vi "Tag Settings Window.vi"(8 "Error In":errorcluster, 11 "Database Connection":refnum<k7>) -> (0 "Error Out":errorcluster)   [LabVIEW 2019]
panel:
  in  "Link Tag Button":bool
  in  "Edit Tag Button":bool
  in  "Remove Tag Button":bool
  in  "Add Tag Button":bool
  in  "Exit Button":bool
  in  "Tag List":i32(listbox) caption="Tags for Device USB-6008-1:"
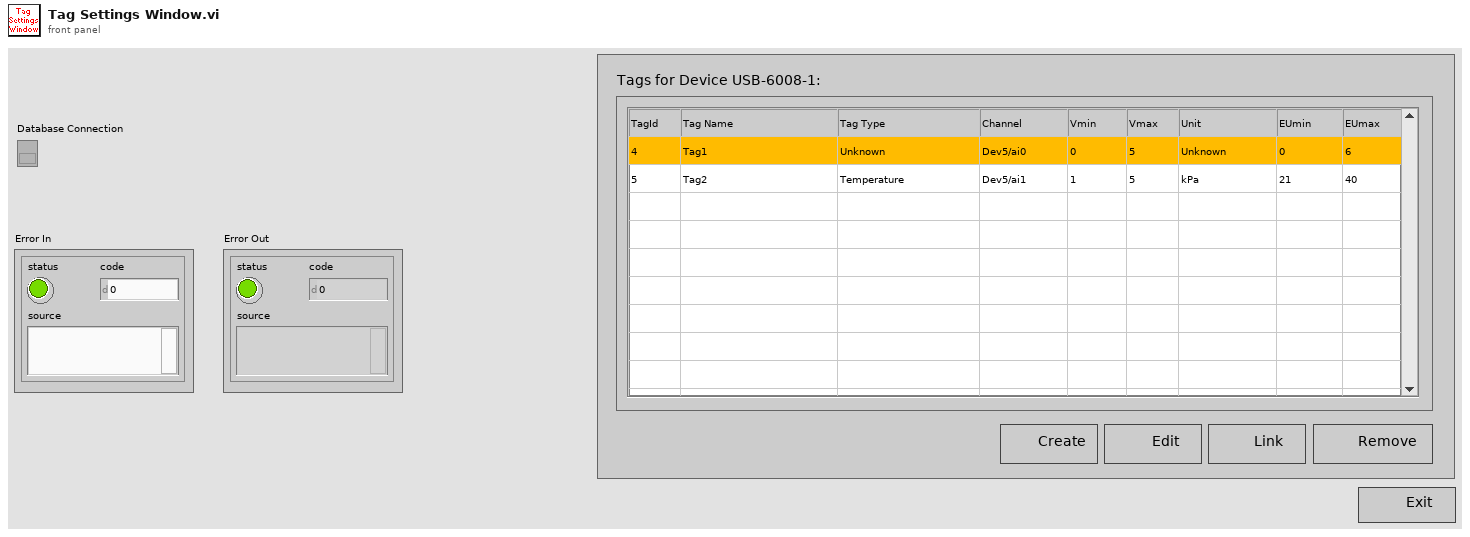
[diagram p1: front panel]
types:
  T1 = typedef "Device Settings.ctl" = cluster{"Device Type":string, "Device Name":string, "DAQmx Name":tag, "Terminal Wiring":i32}
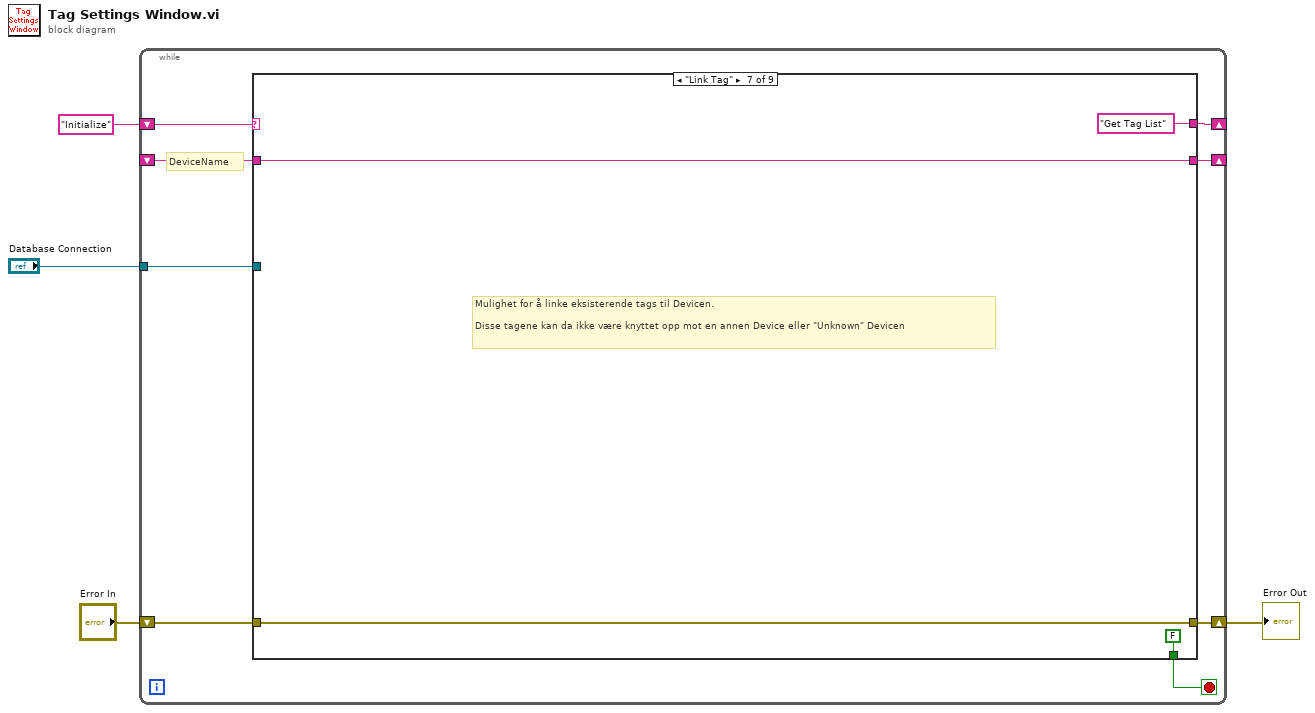
[diagram p0: block diagram]
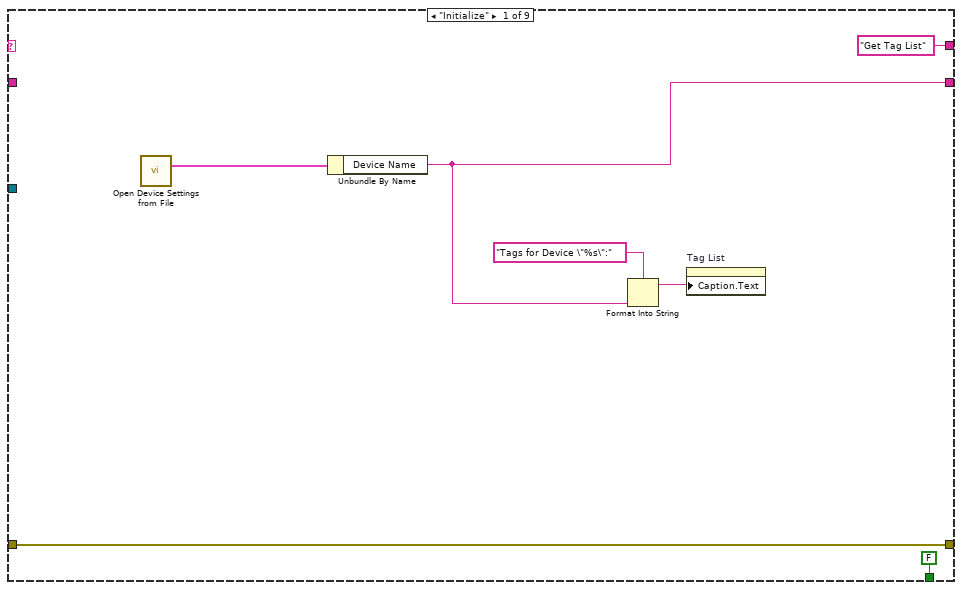
[diagram p2: hidden frame]
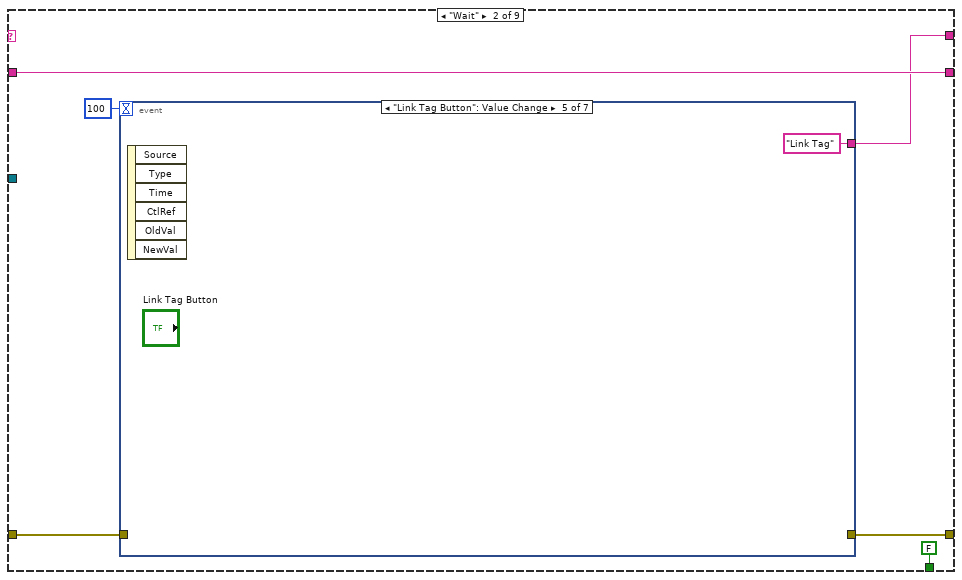
[diagram p3: hidden frame]
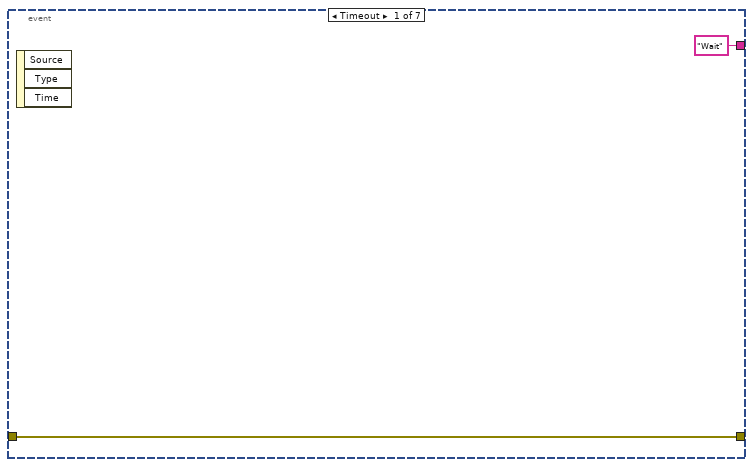
[diagram p4: hidden frame]
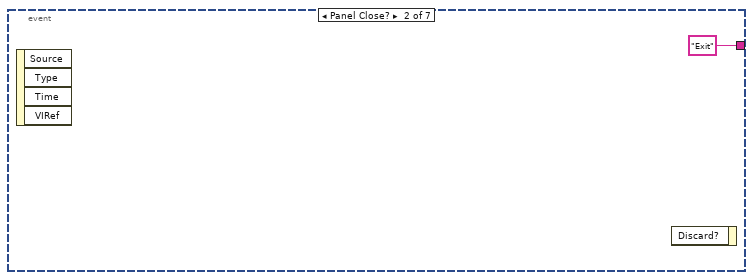
[diagram p5: hidden frame]
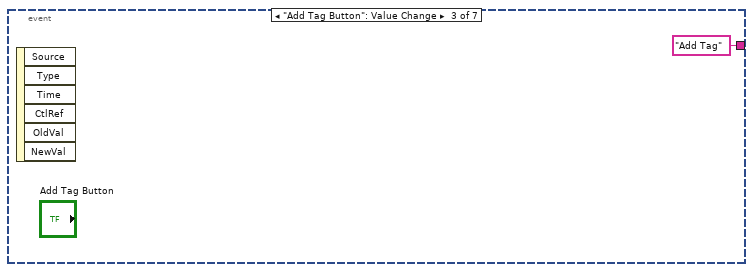
[diagram p6: hidden frame]
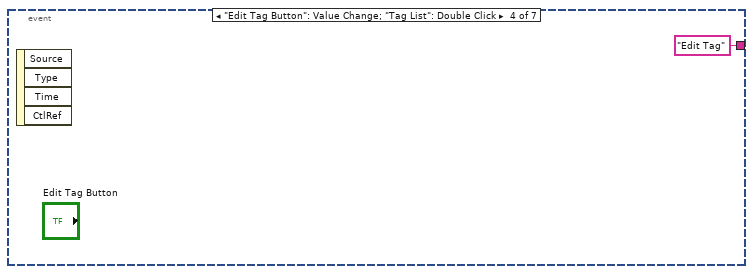
[diagram p7: hidden frame]
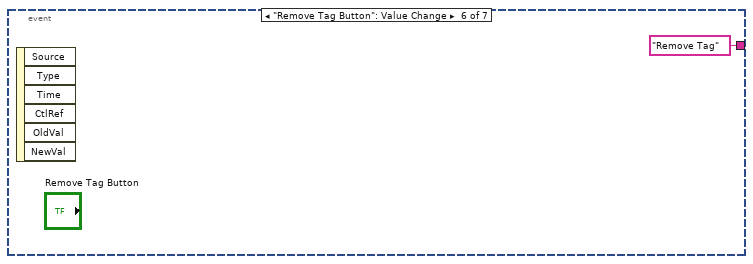
[diagram p8: hidden frame]
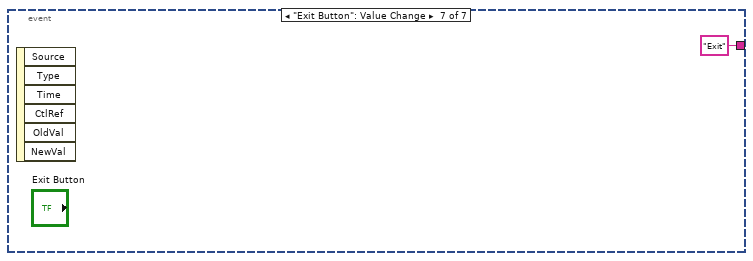
[diagram p9: hidden frame]
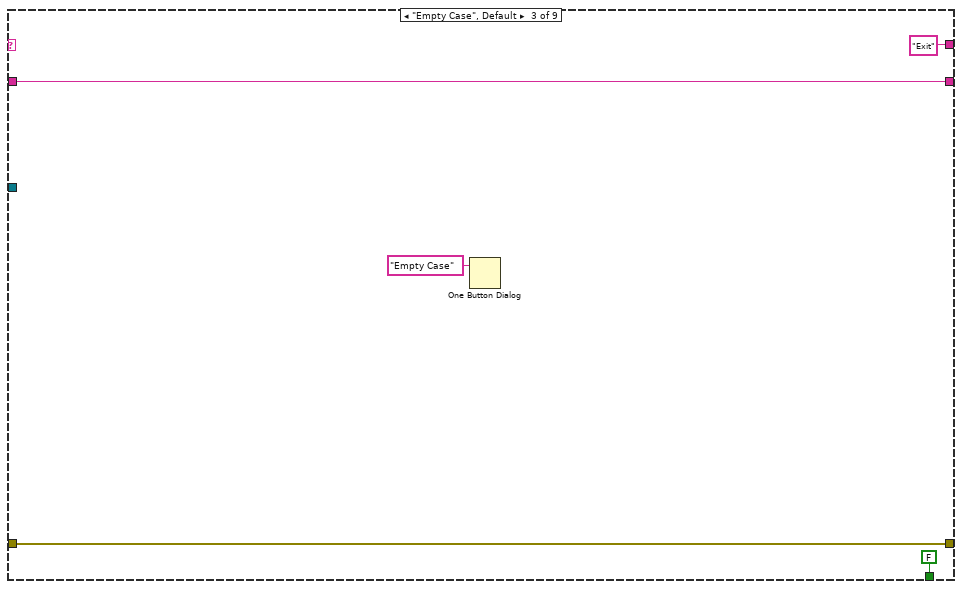
[diagram p10: hidden frame]
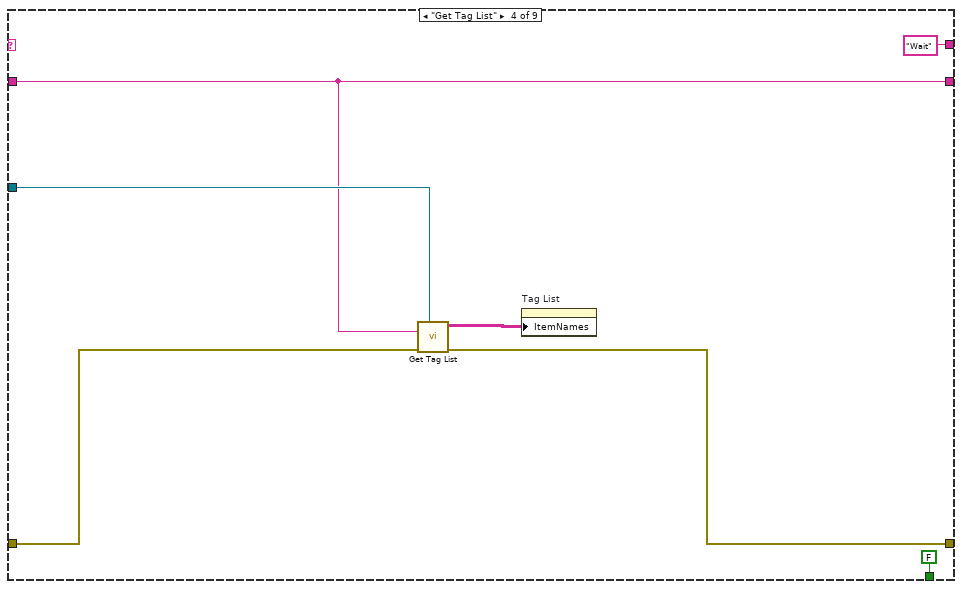
[diagram p11: hidden frame]
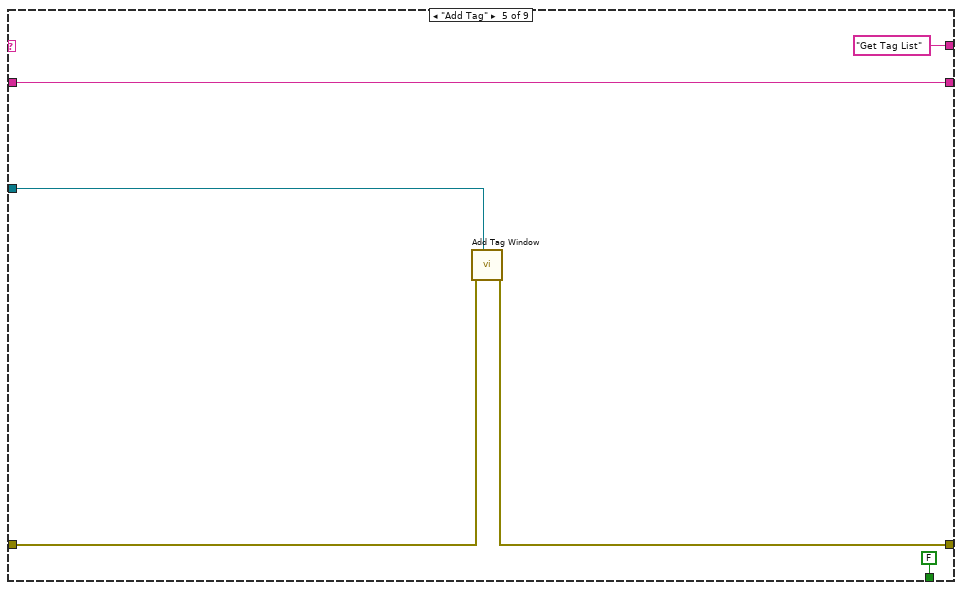
[diagram p12: hidden frame]
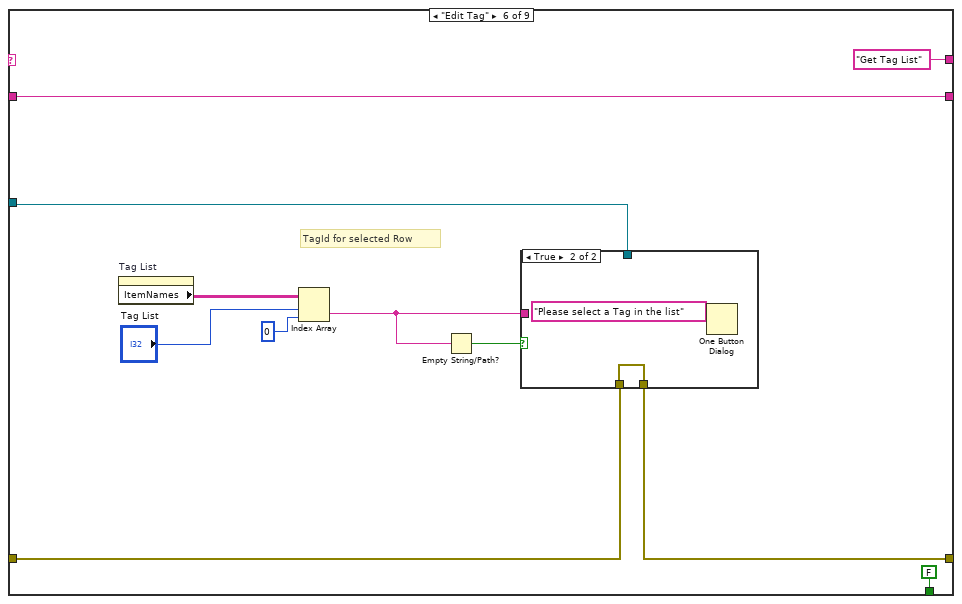
[diagram p13: hidden frame]
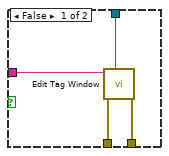
[diagram p14: hidden frame]
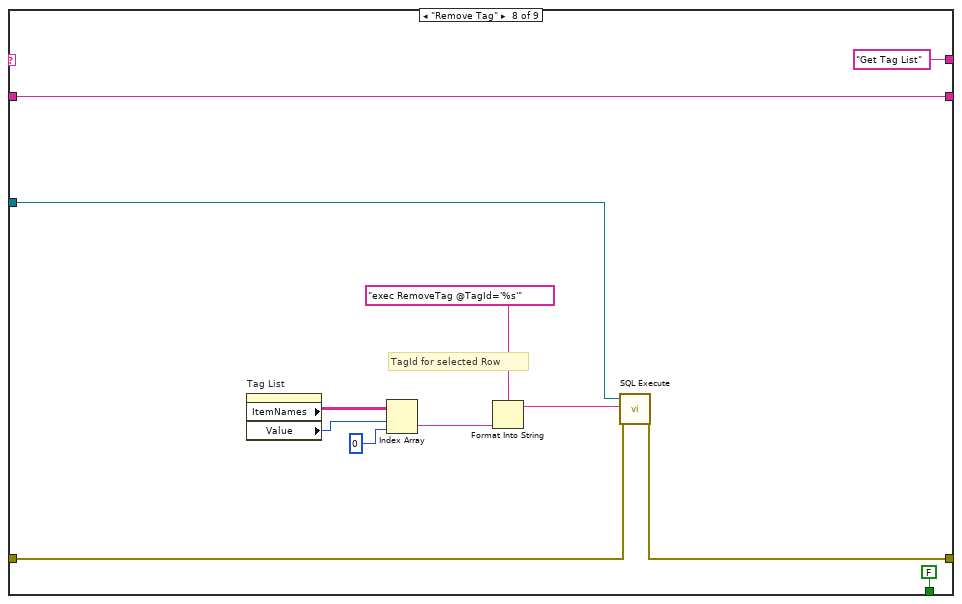
[diagram p15: hidden frame]
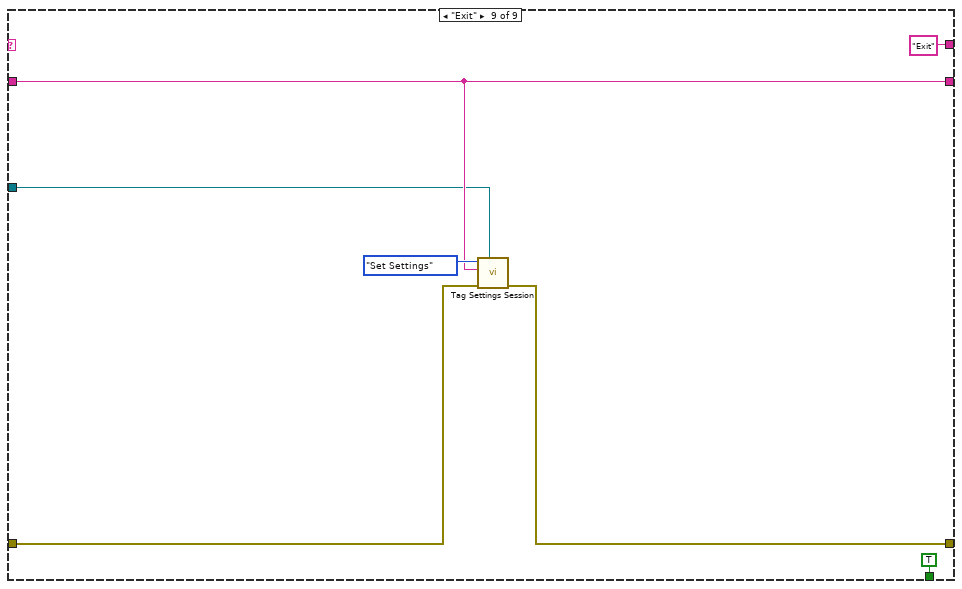
[diagram p16: hidden frame]
diagram:
  n1 = while {
    shift-right: [w8] -> _
    shift-left: "Initialize" ("key") -> [w12]
    shift-right: [w9] -> _
    shift-left: _ -> [w11]
    shift-right: [w6] -> w2
    shift-left: "Error In" -> [w10]
    tunnel: "Database Connection" -> [w5]
    stop <- w7 stop-if-true
    # "DeviceName"
    n2 = case shown="\"Link Tag\"" w12 {
      tunnel: w11 -> [_ w24 w35 w40 w49 w60 w70 w82 w86]
      tunnel: w10 -> [w17 w21 w36 w39 w48 w57 w69 w80 w88]
      tunnel: [w14 w24 w35 w40 w49 w60 w70 w82 w86] -> w9
      tunnel: ["Get Tag List" ("key") w23 "Exit" ("key") "Wait" ("key") "Get Tag List" ("key") "Get Tag List" ("key") "Get Tag List" ("key") "Get Tag List" ("key") "Exit" ("key")] -> w8
      tunnel: [FALSE FALSE FALSE FALSE FALSE FALSE FALSE FALSE TRUE] -> w7
      tunnel: [w17 w20 w36 w42 w47 w56 w69 w79 w87] -> w6
      tunnel: w5 -> [_ _ _ w43 w46 w58 _ w81 w85]
      frame "Initialize" {
        n3 = call "Open Device Settings from File.vi"() -> ("Device Settings"=w16:T1)  [unwired: 14 in, 1 out]
        n4 = Unbundle By Name(w16) -> ("Device Name"=w14:string)
        n5 = Format Into String(format string="Tags for Device \"%s\":", w14) -> (resulting string=w13:string)  [unwired: 2 in, 1 out]
        n6 = property on="Tag List" class="MCListbox (strict)"("Caption.Text"=w13) -> ()  [unwired: 2 in, 2 out]
      }
      frame "Wait" {
        n7 = event shown="[4] \"Link Tag Button\": Value Change" {
          selector: _ -> [_ _ _ _ _ _ _]
          dyn-events: _ -> [_ _ _ _ _ _ _]
          timeout: 100 -> [_ _ _ _ _ _ _]
          tunnel: ["Wait" ("key") "Exit" ("key") "Add Tag" ("key") "Edit Tag" ("key") "Link Tag" ("key") "Remove Tag" ("key") "Exit" ("key")] -> w23
          tunnel: w21 -> [w26 _ _ _ _ _ _]
          tunnel: [w26 _ _ _ _ _ _] -> w20
          event Timeout {
            n8 = event-data() -> ()  [unwired: 1 in, 3 out]
          }
          event Panel Close? {
            n9 = event-data() -> ()  [unwired: 1 in, 4 out]
            n10 = event-data() -> ()  [unwired: 2 in, 1 out]
          }
          event "Add Tag Button": Value Change {
            n11 = event-data() -> ()  [unwired: 1 in, 6 out]
          }
          event "Edit Tag Button": Value Change; "Tag List": Double Click {
            n12 = event-data() -> ()  [unwired: 1 in, 4 out]
          }
          event "Link Tag Button": Value Change {
            n13 = event-data() -> ()  [unwired: 1 in, 6 out]
          }
          event "Remove Tag Button": Value Change {
            n14 = event-data() -> ()  [unwired: 1 in, 6 out]
          }
          event "Exit Button": Value Change {
            n15 = event-data() -> ()  [unwired: 1 in, 6 out]
          }
        }
      }
      frame "Empty Case", Default {
        n16 = One Button Dialog(message="Empty Case") -> ()  [unwired: 1 in, 1 out]
      }
      frame "Get Tag List" {
        n17 = call "Get Tag List.vi"("Database Connection"=w43, "Error In"=w39, "DeviceName"=w40) -> ("Error Out"=w42:errorcluster, "Tag List"=w41:string[][])  [unwired: 7 in]
        n18 = property on="Tag List" class="MCListbox (strict)"("ItemNames"=w41) -> ()  [unwired: 2 in, 2 out]
      }
      frame "Add Tag" {
        n19 = call "Add Tag Window.vi"("Database Connection"=w46, "Error In"=w48) -> ("Error Out"=w47:errorcluster)  [unwired: 9 in]
      }
      frame "Edit Tag" {
        # "TagId for selected Row"
        n20 = property on="Tag List" class="MCListbox (strict)"() -> ("ItemNames"=w59:string[][])  [unwired: 2 in, 2 out]
        n21 = Index Array "Index Array"(array=w59, index (row)="Tag List", index (col)=0 ("index (row)")) -> (element=w53:string)
        n22 = Empty String/Path?(string/path=w53) -> (empty?=w52:bool)
        n23 = case shown="True" w52 {
          tunnel: w58 -> [w66 _]
          tunnel: w57 -> [w65 w68]
          tunnel: [w64 w68] -> w56
          tunnel: w53 -> [w63 _]
          frame False {
            n24 = call "Edit Tag Window.vi"("Database Connection"=w66, "Error In"=w65, "TagId"=w63) -> ("Error Out"=w64:errorcluster)  [unwired: 8 in]
          }
          frame True {
            n25 = One Button Dialog(message="Please select a Tag in the list") -> ()  [unwired: 1 in, 1 out]
          }
        }
      }
      frame "Link Tag" {
        # "Mulighet for å linke eksisterende tags til Devicen.\n\nDisse tagene kan da ikke være knyttet opp mot en annen Device eller \"Unknown\" Devicen"
      }
      frame "Remove Tag" {
        # "TagId for selected Row"
        n26 = property on="Tag List" class="MCListbox (strict)"() -> ("ItemNames"=w77:string[][], "Value"=w76:i32)  [unwired: 2 in, 2 out]
        n27 = Index Array "Index Array"(array=w77, index (row)=w76, index (col)=0 ("index (row)")) -> (element=w75:string)
        n28 = Format Into String "Format Into String"(format string="exec RemoveTag @TagId='%s'", w75) -> (resulting string=w73:string)  [unwired: 2 in, 1 out]
        n29 = call <vilib>:"SQL Execute.vi"("Connection In"=w81, "SQL Query"=w73, "Error in (no error)"=w80) -> ("Error out"=w79:errorcluster)  [unwired: 15 in, 1 out]
      }
      frame "Exit" {
        n30 = call "Tag Settings Session.vi"("Database Connection"=w85, "Error In"=w88, "DeviceName"=w86, "Type"=enum16{"Set Settings", "Get Settings"}."Set Settings") -> ("Error Out"=w87:errorcluster)  [unwired: 6 in, 1 out]
      }
    }
  }
  "Error Out" <- w2
